vi "CVSUI.vi"() -> ()   [LabVIEW 2013, in "PLTarget CVS.lvclass"]
uses:
  PLTarget CVS.lvclass
  Configuration Editor/subVIs/Additional Files Array.ctl
  Configuration Editor/Classes/TBM Configuration Node/deployment configuration.ctl
  <vilib>/NI/Tag Bus Module Framework/root configuration/Target Types.ctl
  <vilib>/NI/Configuration Framework/Node/NodeRef.ctl
  <vilib>/NI/Configuration Framework/Node/NISE_CEF_Node.lvclass
  <vilib>/NI/AMC/Message Queue.ctl
  <vilib>/NI/AMC/Message.ctl
  <vilib>/NI/Tools/Keyed Array/KeyedArray.ctl
  <vilib>/NI/Configuration Framework/Node/UserEventRef.ctl
  <vilib>/NI/Configuration Framework/Controls/EventCluster.ctl
  <vilib>/NI/Configuration Framework/Node/RefreshUIEvent.ctl
  <vilib>/NI/Configuration Framework/Node/CacheState.ctl
  <vilib>/NI/Configuration Framework/Node/StopEvent.ctl
  <vilib>/NI/Configuration Framework/Node/NodeChangeEvent.ctl
  <vilib>/Utility/miscctls.llb/LVPositionTypeDef.ctl
  Configuration Editor/Classes/Targets/Targets.lvclass/Targets.ctl
  PLTarget CVS.lvclass/PLTarget CVS.ctl
  Framework Configuration Classes/target configuration/PL_Target Configuration.lvclass/PL_Target Configuration.ctl
  <vilib>/NI/Configuration Framework/serializable node/NISE_CEF_serializable node.lvclass
  <vilib>/NI/Tag Bus Module Framework/root configuration/TBM configuration.lvclass
  Configuration Editor/Classes/Targets/Write additional files.vi
  Configuration Editor/Classes/Targets/Read additional files.vi
  <vilib>/NI/Configuration Framework/serializable configuration/set alias.vi
  <vilib>/NI/Configuration Framework/serializable configuration/get alias.vi
  <vilib>/NI/Configuration Framework/serializable configuration/NISE_CEF_serializable configuration.lvclass
  Framework Configuration Classes/target configuration/PL_Target Configuration.lvclass
  Configuration Editor/Classes/Targets/Targets.lvclass
  <vilib>/NI/DCAF UI Toolkit/Controls/DCAF UI Elements.lvlib
  <vilib>/NI/Tools/Keyed Array/Tools_KeyedArray.lvlib
  <vilib>/NI/AMC/AMC.lvlib
  <vilib>/NI/Configuration Framework/NISE_CEF_TreeControl.lvlib
  Configuration Editor/Classes/TBM Configuration Node/TBM Configuration Node.lvclass
panel:
  in  "Top Level Tab Control":enum32{"Configuration", "Additional Files"}(tab)
  in  "Target Type":T1=enum."Linux RT ARM"
  in  "IP":string
  in  "Name":string
  in  "Includes file path":path
  in  "path to deploy on target relative to root (c:\\ or /home/lvuser/)":path
  in  "generate includes file":bool
  in  "load bitfile":bool
  in  "RIO FPGA":string="RIO0"
  in  "bitfile path on target relative to root (c:\\ or /home/lvuser/)":path
  in  "Local Bitfile Path":path
  in  "Additional Files":T2
  in  "node change":T4
  in  "stop event":T5
  in  "cache state":T6
  in  "refresh UI":T7
  in  "open fp?":bool=TRUE
  in  "user event":T8
  in  "main queue":T9
  in  "node ref":T10
  # "Target Information"
  # "Deployment Settings"
  # "FPGA Settings"
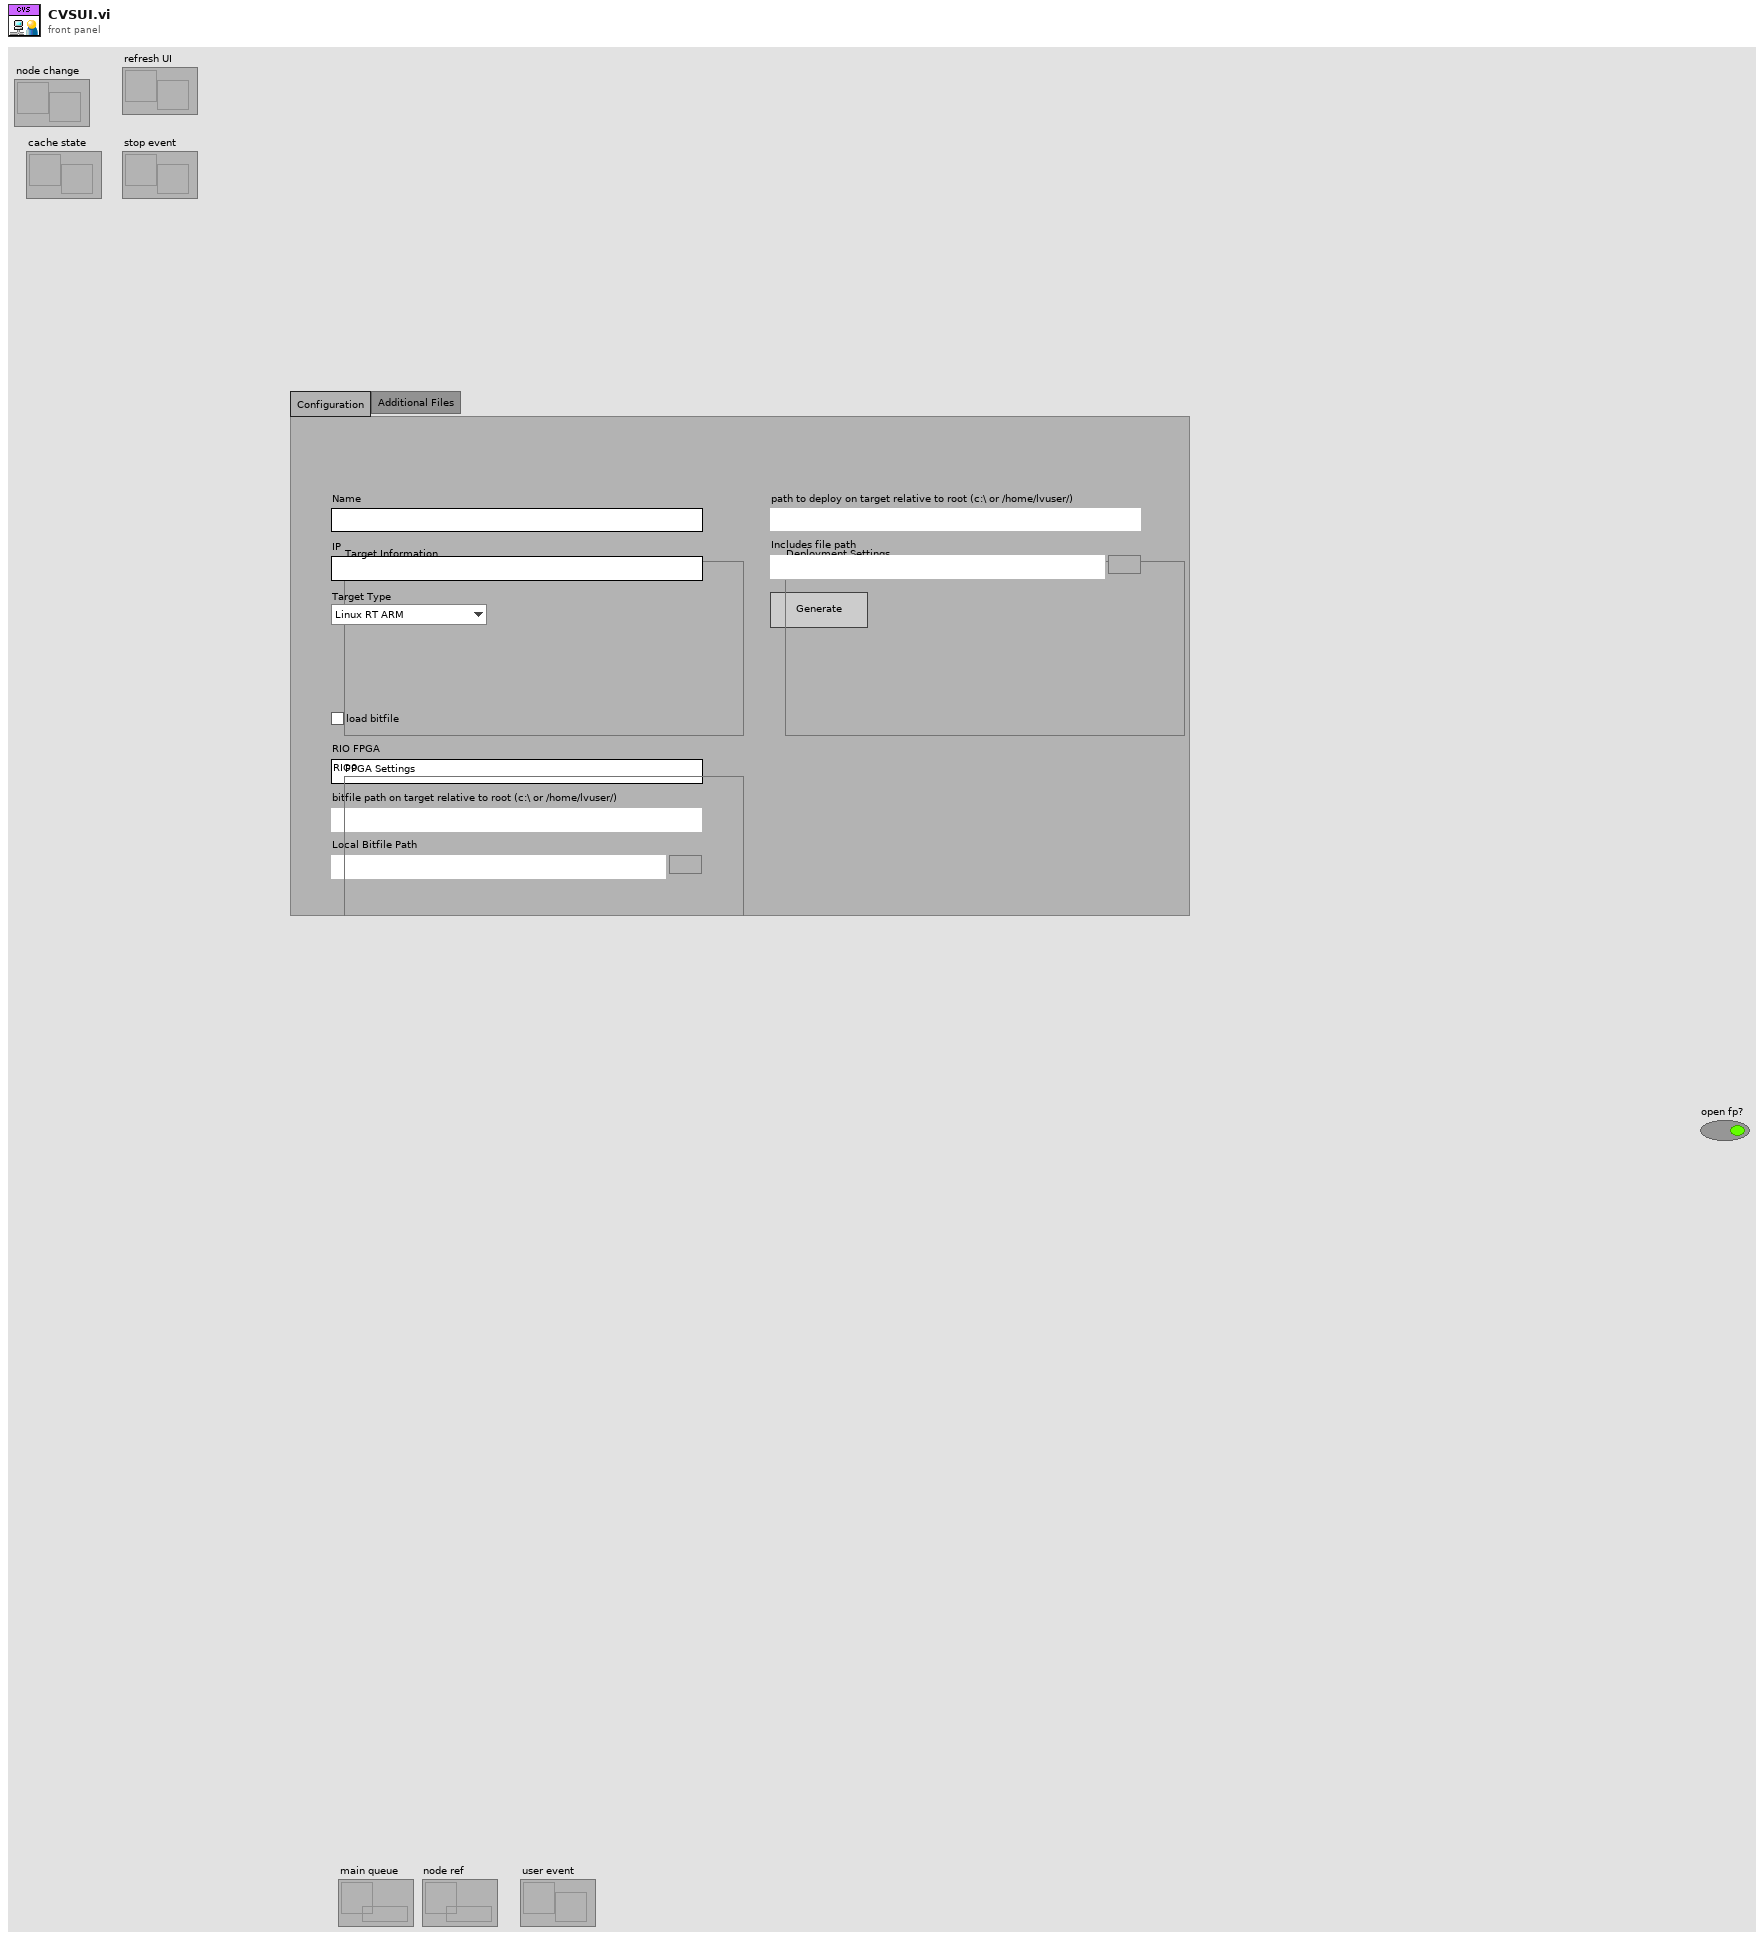
[diagram p1: front panel]
types:
  T1 = typedef "TBM configuration.lvclass/Target Types.ctl" = enum16{"Windows", "Mac", "Linux", "Linux RT ARM", "VxWorks", "Pharlap", "Other", "Linux RT x64"}
  T2 = typedef "Additional Files Array.ctl" = T3[]
  T3 = typedef "PL Framework Configuration Tool.lvlib/TBM Configuration Node.lvclass/deployment configuration.ctl" = cluster{"local path":path, "remote path (relative to root)":path}
  T4 = typedef "NISE_CEF_Node.lvclass/NodeChangeEvent.ctl" = refnum<user-event>
  T5 = typedef "NISE_CEF_Node.lvclass/StopEvent.ctl" = refnum<user-event>
  T6 = typedef "NISE_CEF_Node.lvclass/CacheState.ctl" = refnum<user-event>
  T7 = typedef "NISE_CEF_Node.lvclass/RefreshUIEvent.ctl" = refnum<user-event>
  T8 = typedef "NISE_CEF_Node.lvclass/UserEventRef.ctl" = refnum<user-event>
  T9 = typedef "AMC.lvlib/Message Queue.ctl" = refnum<queue>
  T10 = typedef "NISE_CEF_Node.lvclass/NodeRef.ctl" = refnum<data-value>
  T11 = typedef "LVPositionTypeDef.ctl" = cluster{"Left":i32, "Top":i32}
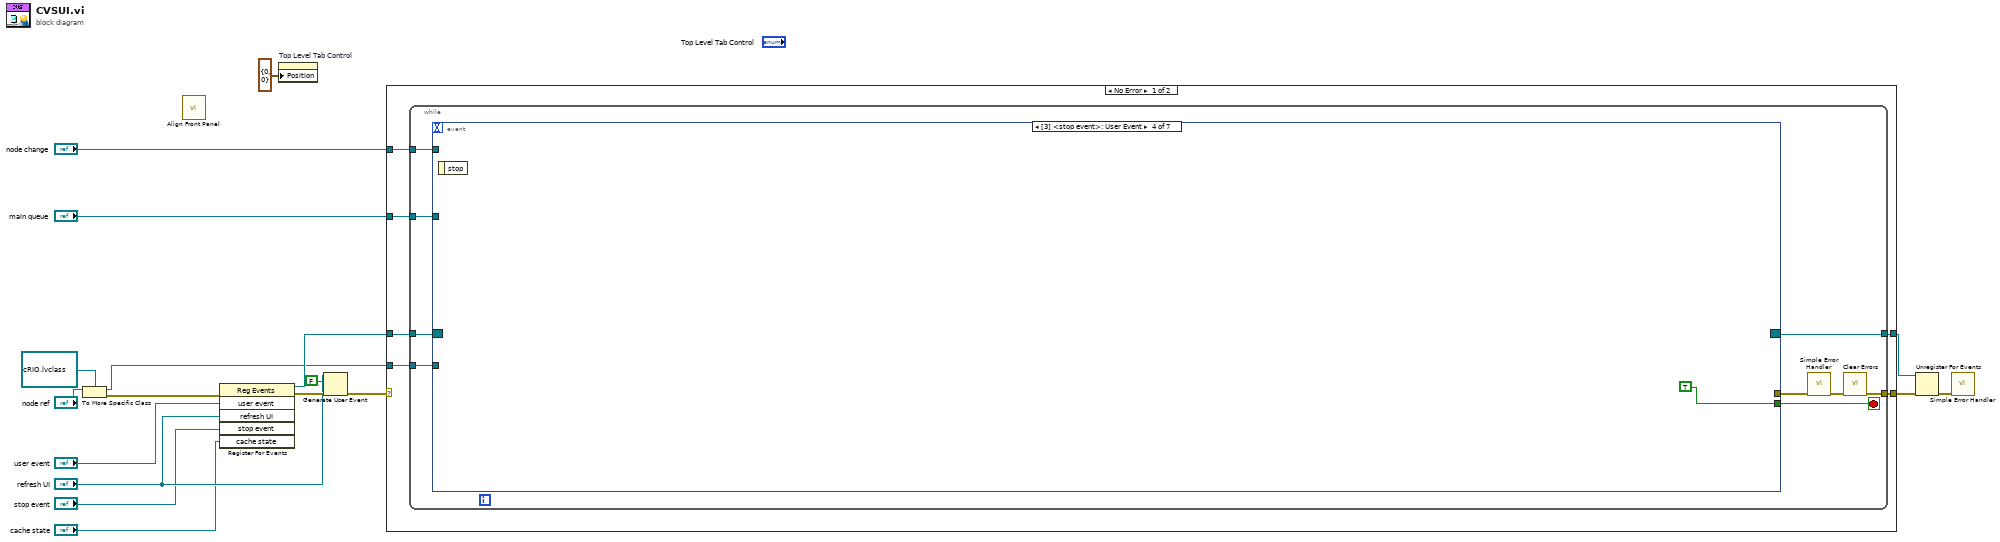
[diagram p0: block diagram]
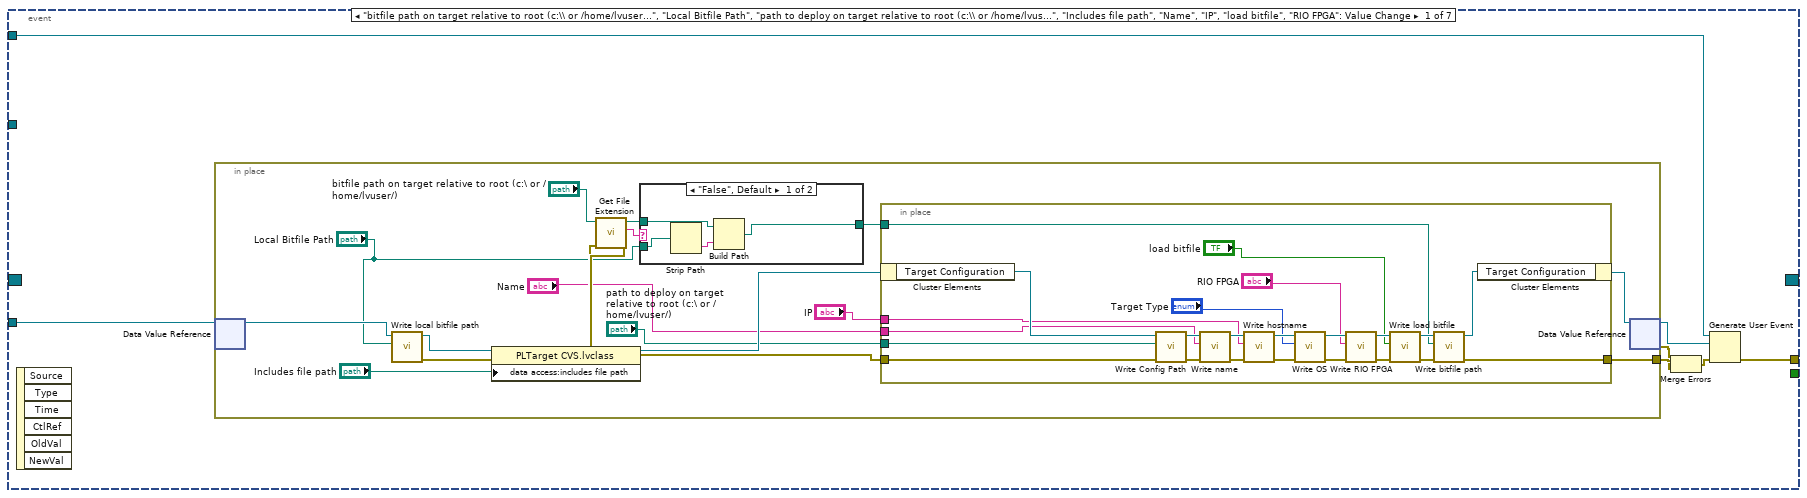
[diagram p2: hidden frame]
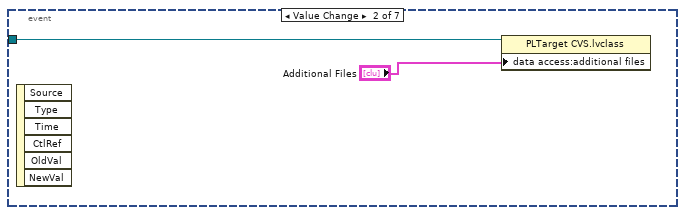
[diagram p4: hidden frame]
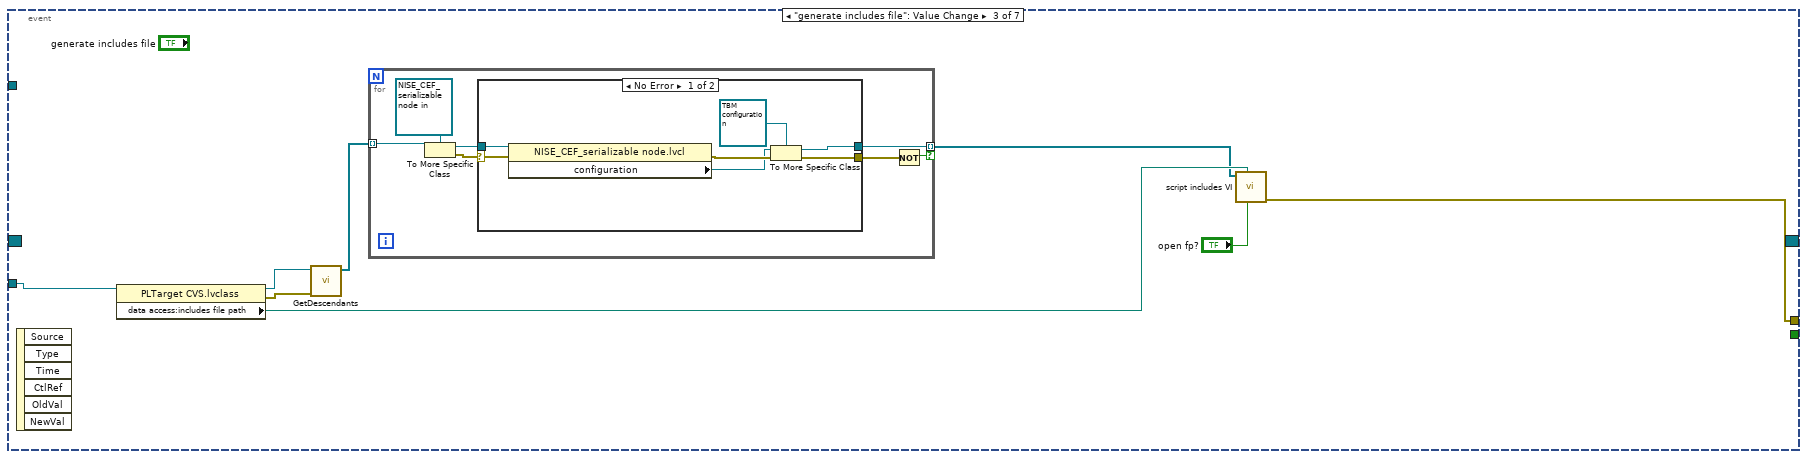
[diagram p5: hidden frame]
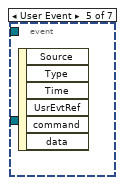
[diagram p7: hidden frame]
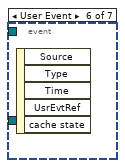
[diagram p8: hidden frame]
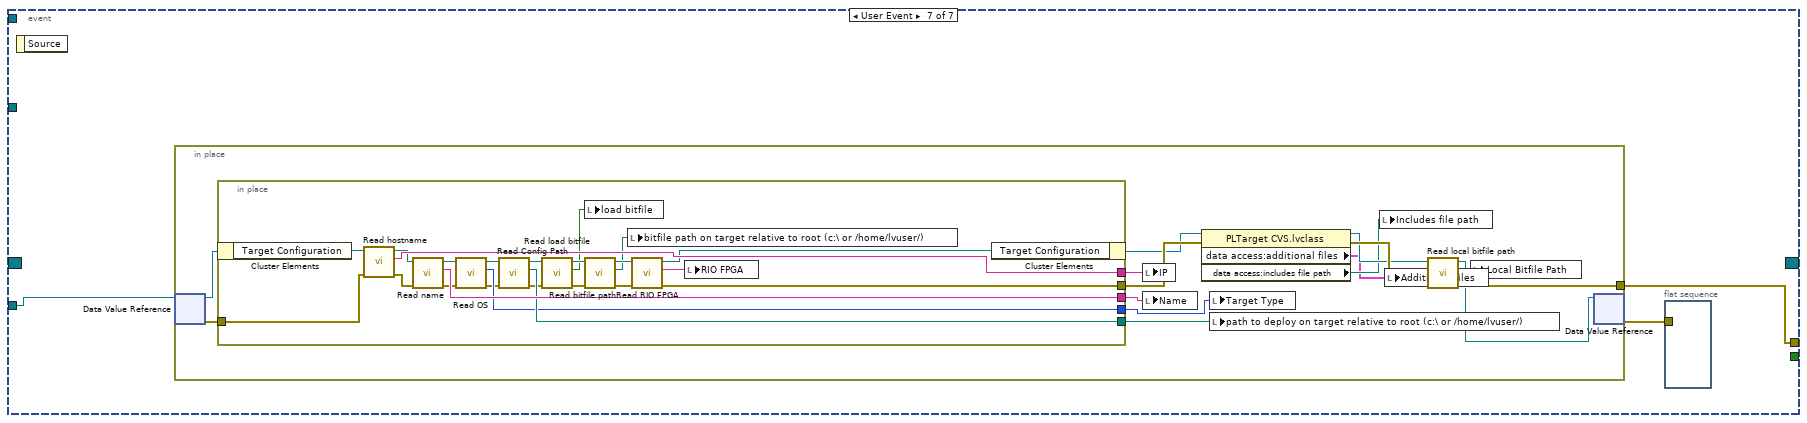
[diagram p9: hidden frame]
diagram:
  n1 = To More Specific Class(target class=refnum<data-value> refnum ("data value reference"), reference="node ref") -> (specific class reference=w5:refnum<data-value>, error out=w6:errorcluster)  [unwired: 1 in]
  n2 = call <vilib>:"Align Front Panel.vi"() -> ()  [unwired: 10 in, 2 out]
  n3 = register-events(error in=w6, "user event", "refresh UI", "stop event", "cache state") -> (reference out=w16:refnum<event-registration>, error out=w13:errorcluster)  [unwired: 1 in]
  n4 = property on="Top Level Tab Control" class="TabCtl (strict)"("Position"=T11 {"Left"=0, "Top"=0}) -> ()  [unwired: 2 in, 2 out]
  n5 = Generate User Event(user event="refresh UI", event data cluster=FALSE ("event data"), error in=w13) -> (error out=w7:errorcluster)  [unwired: 1 in, 1 out]
  n6 = case shown="No Error" w7 {
    selector: w7 -> [_ w153]
    tunnel: w5 -> [w24 _]
    tunnel: "main queue" -> [w23 _]
    tunnel: w16 -> [w22 w154]
    tunnel: [w21 w154] -> w15
    tunnel: [w20 w153] -> w14
    tunnel: "node change" -> [w19 _]
    frame No Error {
      n7 = while {
        tunnel: w24 -> [w33]
        tunnel: w23 -> [w32]
        tunnel: w22 -> [w31]
        tunnel: [w30] -> w21
        tunnel: [w26] -> w20
        tunnel: w19 -> [w25]
        stop <- w29 stop-if-true
        n8 = event shown="[3] <stop event>: User Event" {
          selector: w31 -> [_ _ _ _ _ _ _]
          dyn-events: [_ _ _ _ _ _ _] -> w30
          timeout: _ -> [_ _ _ _ _ _ _]
          tunnel: w33 -> [w40 w87 w95 _ _ _ w114]
          tunnel: w32 -> [_ _ _ _ _ _ _]
          tunnel: [_ _ _ TRUE _ _ _] -> w29
          tunnel: [w38 _ w92 _ _ _ w113] -> w28
          tunnel: w25 -> [w37 _ _ _ _ _ _]
          event "bitfile path on target relative to root (c:\\ or /home/lvuser/)", "Local Bitfile Path", "path to deploy on target relative to root (c:\\ or /home/lvuser/)", "Includes file path", "Name", "IP", "load bitfile", "RIO FPGA": Value Change {
            n9 = event-data() -> ()  [unwired: 1 in, 6 out]
            n10 = in-place {
              in-place-border: [w56] -> w39
              n11 = in-place-dvr #1(w40) -> (w55:refnum<class "PLTarget CVS.lvclass">)  [unwired: 1 out]
              n12 = call "Write local bitfile path.vi"("bitfile path"="Local Bitfile Path", "Targets in"=w55) -> ("error out"=w51:errorcluster, "Targets out"=w48:refnum<class "PLTarget CVS.lvclass">)  [unwired: 8 in]
              n13 = property class="PLTarget CVS.lvclass"(reference=w48, error in=w51, "data access:includes file path"="Includes file path") -> (reference out=w47:refnum<class "PLTarget CVS.lvclass">, error out=w49:errorcluster)
              n14 = call <vilib>:"Get File Extension.vi"("error in (no error)"=w49, "file"="bitfile path on target relative to root (c:\\ or /home/lvuser/)") -> ("error out"=w50:errorcluster, "lowercase file extension"=w54:string, "dup file"=w52:path)  [unwired: 6 in, 1 out]
              n15 = case shown="\"False\", Default" w54 {
                tunnel: [w60 w62] -> w53
                tunnel: w52 -> [w61 w62]
                tunnel: "Local Bitfile Path" -> [w58 _]
                frame "False", Default {
                  n16 = Strip Path(path=w58) -> (name=w59:string)  [unwired: 1 out]
                  n17 = Build Path(base path=w61, name or relative path=w59) -> (appended path=w60:path)
                }
                frame "lvbit", "lvbitx" {
                }
              }
              n18 = in-place {
                in-place-border: "path to deploy on target relative to root (c:\\ or /home/lvuser/)" -> [w84]
                in-place-border: "IP" -> [w81]
                in-place-border: "Name" -> [w80]
                in-place-border: w50 -> [w68]
                in-place-border: [w67] -> w56
                in-place-border: w53 -> [w66]
                n19 = in-place-cluster #2(w47) -> ("Target Configuration"=w85:refnum<class "PL_Target Configuration.lvclass">)
                n20 = call "Write Config Path.vi"("error in"=w68, "Config Path"=w84, "PL_Local Target Configuration in"=w85) -> ("error out"=w72:errorcluster, "PL_Local Target Configuration out"=w83:refnum<class "PL_Target Configuration.lvclass">)  [unwired: 7 in]
                n21 = call "Write name.vi"("error in"=w72, "name"=w80, "PL_Local Target Configuration in"=w83) -> ("error out"=w71:errorcluster, "PL_Local Target Configuration out"=w82:refnum<class "PL_Target Configuration.lvclass">)  [unwired: 7 in]
                n22 = call "Write hostname.vi"("error in"=w71, "hostname"=w81, "PL_Target Configuration in"=w82) -> ("error out"=w70:errorcluster, "PL_Target Configuration out"=w79:refnum<class "PL_Target Configuration.lvclass">)  [unwired: 7 in]
                n23 = call "Write OS.vi"("error in"=w70, "Target Types"="Target Type", "PL_Target Configuration in"=w79) -> ("error out"=w69:errorcluster, "PL_Target Configuration out"=w74:refnum<class "PL_Target Configuration.lvclass">)  [unwired: 7 in]
                n24 = call "Write RIO FPGA.vi"("error in"=w69, "RIO FPGA"="RIO FPGA", "PL_Target Configuration in"=w74) -> ("error out"=w76:errorcluster, "PL_Target Configuration out"=w75:refnum<class "PL_Target Configuration.lvclass">)  [unwired: 7 in]
                n25 = call "Write load bitfile.vi"("error in"=w76, "load bitfile"="load bitfile", "PL_Target Configuration in"=w75) -> ("error out"=w78:errorcluster, "PL_Target Configuration out"=w77:refnum<class "PL_Target Configuration.lvclass">)  [unwired: 7 in]
                n26 = call "Write bitfile path.vi"("error in"=w78, "bitfile path"=w66, "PL_Target Configuration in"=w77) -> ("error out"=w67:errorcluster, "PL_Target Configuration out"=w73:refnum<class "PL_Target Configuration.lvclass">)  [unwired: 7 in]
                n27 = in-place-cluster #2("Target Configuration"=w73) -> (w57:refnum<class "PLTarget CVS.lvclass">)
              }
              n28 = in-place-dvr #1(w57) -> (w36:refnum<data-value>, w34:errorcluster)
            }
            n29 = Merge Errors(w39, w34) -> (w35:errorcluster)
            n30 = Generate User Event(user event=w37, event data cluster=w36, error in=w35) -> (error out=w38:errorcluster)  [unwired: 1 in, 1 out]
          }
          event Value Change {
            n31 = event-data() -> ()  [unwired: 1 in, 6 out]
            n32 = property class="PLTarget CVS.lvclass"(reference=w87, "data access:additional files"="Additional Files") -> ()  [unwired: 1 in, 2 out]
          }
          event "generate includes file": Value Change {
            n33 = event-data() -> ()  [unwired: 1 in, 6 out]
            n34 = property class="PLTarget CVS.lvclass"(reference=w95) -> (reference out=w90:refnum<data-value>, error out=w91:errorcluster, "data access:includes file path"=w93:path)  [unwired: 1 in]
            n35 = call <vilib>:"GetDescendants.vi"("error in"=w91, "node in"=w90) -> ("descendants"=w89:refnum<data-value>[])  [unwired: 8 in, 1 out]
            n36 = for {
              tunnel: w89 -> [w102] mode=indexing
              tunnel: [w98] -> w88 mode=indexing if=w96
              n37 = To More Specific Class(target class=refnum<data-value> refnum, reference=w102) -> (specific class reference=w99:refnum<data-value>, error out=w100:errorcluster)  [unwired: 1 in]
              n38 = case shown="No Error" w100 {
                selector: w100 -> [w108 w110]
                tunnel: w99 -> [w109 _]
                tunnel: [w103 _] -> w98
                tunnel: [w106 w110] -> w97
                frame No Error {
                  n39 = property class="NISE_CEF_serializable node.lvcl"(reference=w109, error in=w108) -> (error out=w107:errorcluster, "configuration"=w105:refnum<class "NISE_CEF_serializable configuration.lvclass">)  [unwired: 1 out]
                  n40 = To More Specific Class(target class=refnum<class "TBM configuration.lvclass"> refnum ("configuration"), reference=w105, error in=w107) -> (specific class reference=w103:refnum<class "TBM configuration.lvclass">, error out=w106:errorcluster)
                }
                frame Error {
                }
              }
              n41 = Not(x=w97) -> (.not. x?=w96:bool)
            }
            n42 = call "script includes VI.vi"("open fp?"="open fp?", "vi path (blank=new)"=w93, "cfg objects"=w88) -> ("error out"=w92:errorcluster)  [unwired: 8 in]
          }
          event User Event {
            n43 = event-data() -> ()  [unwired: 1 in, 1 out]
          }
          event User Event {
            n44 = event-data() -> ()  [unwired: 1 in, 6 out]
          }
          event User Event {
            n45 = event-data() -> ()  [unwired: 1 in, 5 out]
          }
          event User Event {
            n46 = event-data() -> ()  [unwired: 1 in, 1 out]
            n47 = in-place {
              in-place-border: [w122] -> w113
              n48 = in-place-dvr #3(w114) -> (w126:refnum<class "PLTarget CVS.lvclass">, w124:errorcluster)
              n49 = in-place {
                in-place-border: [w152] -> w129
                in-place-border: [w147] -> w127
                in-place-border: [w151] -> w128
                in-place-border: [w145] -> w125
                in-place-border: w124 -> [w134]
                in-place-border: [w133] -> w123
                n50 = in-place-cluster #4(w126) -> ("Target Configuration"=w148:refnum<class "PL_Target Configuration.lvclass">)
                n51 = call "Read hostname.vi"("error in"=w134, "PL_Target Configuration in"=w148) -> ("error out"=w144:errorcluster, "hostname"=w151:string, "PL_Target Configuration out"=w149:refnum<class "PL_Target Configuration.lvclass">)  [unwired: 7 in]
                n52 = call "Read name.vi"("error in"=w144, "PL_Local Target Configuration in"=w149) -> ("error out"=w143:errorcluster, "name"=w152:string, "PL_Local Target Configuration out"=w150:refnum<class "PL_Target Configuration.lvclass">)  [unwired: 7 in]
                n53 = call "Read OS.vi"("error in"=w143, "PL_Target Configuration in"=w150) -> ("error out"=w142:errorcluster, "Target Types"=w145:T1, "PL_Target Configuration out"=w146:refnum<class "PL_Target Configuration.lvclass">)  [unwired: 7 in]
                n54 = call "Read Config Path.vi"("error in"=w142, "PL_Local Target Configuration in"=w146) -> ("error out"=w135:errorcluster, "Config Path"=w147:path, "PL_Local Target Configuration out"=w136:refnum<class "PL_Target Configuration.lvclass">)  [unwired: 7 in]
                n55 = call "Read load bitfile.vi"("error in"=w135, "PL_Target Configuration in"=w136) -> ("error out"=w139:errorcluster, "load bitfile"=w130:bool, "PL_Target Configuration out"=w138:refnum<class "PL_Target Configuration.lvclass">)  [unwired: 7 in]
                n56 = local write "load bitfile"(w130) -> ()
                n57 = call "Read bitfile path.vi"("error in"=w139, "PL_Target Configuration in"=w138) -> ("error out"=w141:errorcluster, "bitfile path"=w131:path, "PL_Target Configuration out"=w140:refnum<class "PL_Target Configuration.lvclass">)  [unwired: 7 in]
                n58 = local write "bitfile path on target relative to root (c:\\ or /home/lvuser/)"(w131) -> ()
                n59 = call "Read RIO FPGA.vi"("error in"=w141, "PL_Target Configuration in"=w140) -> ("error out"=w133:errorcluster, "RIO FPGA"=w132:string, "PL_Target Configuration out"=w137:refnum<class "PL_Target Configuration.lvclass">)  [unwired: 7 in]
                n60 = local write "RIO FPGA"(w132) -> ()
                n61 = in-place-cluster #4("Target Configuration"=w137) -> (w118:refnum<class "PLTarget CVS.lvclass">)
              }
              n62 = local write "IP"(w128) -> ()
              n63 = local write "Name"(w129) -> ()
              n64 = property class="PLTarget CVS.lvclass"(reference=w118, error in=w123) -> (reference out=w117:refnum<class "PLTarget CVS.lvclass">, error out=w119:errorcluster, "data access:additional files"=w115:T3[], "data access:includes file path"=w116:path)
              n65 = local write "Target Type"(w125) -> ()
              n66 = local write "path to deploy on target relative to root (c:\\ or /home/lvuser/)"(w127) -> ()
              n67 = local write "Includes file path"(w116) -> ()
              n68 = local write "Additional Files"(w115) -> ()
              n69 = call "Read local bitfile path.vi"("error in"=w119, "Targets in"=w117) -> ("error out"=w122:errorcluster, "bitfile path"=w120:path, "Targets out"=w121:refnum<class "PLTarget CVS.lvclass">)  [unwired: 7 in]
              n70 = local write "Local Bitfile Path"(w120) -> ()
              n71 = in-place-dvr #3(w121) -> (w112:errorcluster)  [unwired: 1 out]
            }
            n72 = flat-sequence {
              tunnel: w112 -> [_]
              frame #0 {
              }
            }
          }
        }
        n73 = call <vilib>:"Simple Error Handler.vi"("error in (no error)"=w28) -> ("error out"=w27:errorcluster)  [unwired: 4 in, 4 out]
        n74 = call <vilib>:"Clear Errors.vi"("error in (no error)"=w27) -> ("error out"=w26:errorcluster)  [unwired: 6 in]
      }
    }
    frame Error {
    }
  }
  n75 = Unregister For Events(event registration refnum=w15, error in=w14) -> (error out=w4:errorcluster)
  n76 = call <vilib>:"Simple Error Handler.vi"("error in (no error)"=w4) -> ()  [unwired: 4 in, 5 out]
